vi "test_gen_verify.vi"() -> ()   [LabVIEW 2011]
panel:
  out "Components Equal":bool
  out "a2 equal":bool
  out "a1 equal":bool
  out "Components equal":bool
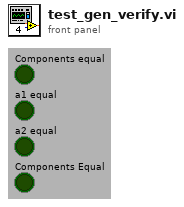
[diagram p1: front panel]
types:
  T1 = cluster{"String":string, "Boolean":bool, "Array":cxt[]}
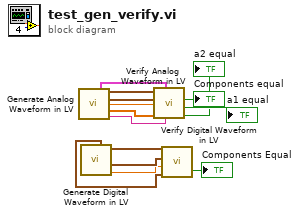
[diagram p0: block diagram]
diagram:
  n1 = call "Generate Analog Waveform in LV.vi"() -> ("a2"=w14:T1, "waveform out"=w11:waveform(dbl), "t0"=w9:timestamp, "dt"=w12:dbl, "Y"=w10:dbl[], "a1"=w13:string)  [unwired: 10 out]
  n2 = call "Generate Digital Waveform in LV.vi"() -> ("Y"=w1:digitaldata, "digital waveform"=w5:digitalwaveform, "t0"=w4:timestamp, "dt"=w2:dbl)  [unwired: 1 in, 2 out]
  n3 = call "Verify Analog Waveform in LV.vi"("a1"=w13, "a2"=w14, "Y"=w10, "dt"=w12, "t0"=w9, "waveform in"=w11) -> ("a2 equal"=→"a2 equal":bool, "a1 equal"=→"a1 equal":bool, "Components equal"=→"Components equal":bool)  [unwired: 1 out]
  n4 = call "Verify Digital Waveform in LV.vi"("Y"=w1, "dt"=w2, "t0"=w4, "digital waveform"=w5) -> ("Components Equal"=→"Components Equal":bool)  [unwired: 1 out]
